vi "UpdateProcNok.vi"(8 "Error In":errorcluster, 11 "Data":variant) -> (0 "Error Out":errorcluster)   [LabVIEW 2023, in "QSM - Alarms.lvlib"]
uses:
  QSM - Alarms.lvlib
  Controls/Message Queue Element Position.ctl
  Controls/State Machine Message.ctl
  SubVIs/Enqueue Message (Single).vi
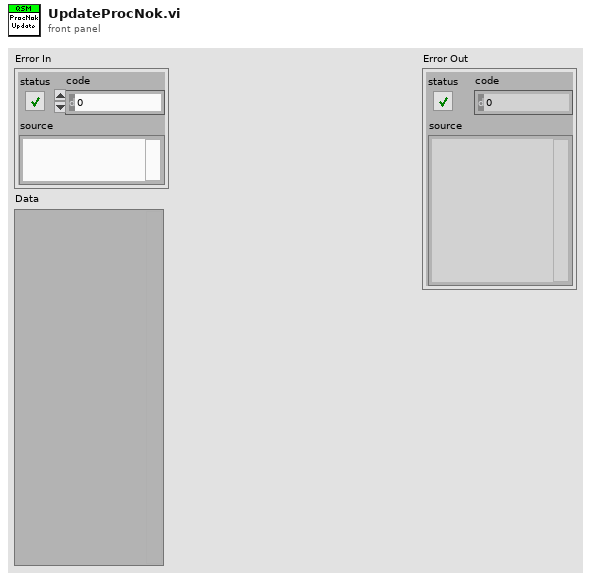
[diagram p1: front panel]
types:
  T1 = typedef "QSM - Alarms.lvlib/State Machine Message.ctl" = enum16{"Initialize", "PROC OK Change", "Get Main PROCNOK", "CLEAR PROC NOK", "ALARM SET", "CLEAR ALARMS", "CHECKS", "Handle Error", "Exit"}
  T2 = typedef "QSM - Alarms.lvlib/Message Queue Element Position.ctl" = enum16{"Front", "Back"}
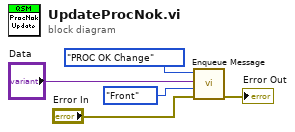
[diagram p0: block diagram]
diagram:
  n1 = call-poly "Enqueue Message.vi"("Error In"="Error In", "Message Position"=Message_Queue_Element_Position."Front", "Data"="Data", "State Machine Message"=State_Machine_Message."PROC OK Change") -> ("Error Out"=→"Error Out":errorcluster)  [unwired: 7 in]
